vi "Button Lower Arm.vi"(7 "Description":string, 8 "Command Info In":T1, 9 "Deadband Value":dbl=0.01, 10 "Duration":dbl, 11 "Setpoint":dbl) -> (0 "Command Info Out":T1)   [LabVIEW 2017]
doc: "This template includes code for deadband comparision to avoid excessive command scheduling. It is particularly useful for joystick-driven commands.\n\nBe sure to right-click and select New from Template and save with a new command name."
uses:
  <vilib>/Rock Robotics/WPI/Framework/Command Status Info.ctl
  <vilib>/Rock Robotics/WPI/Framework/Completion Status.ctl
  <vilib>/Rock Robotics/WPI/Framework/Completion Notifier.ctl
  Implementation/Arm Setpoints.ctl
  Implementation/Arm Operations.ctl
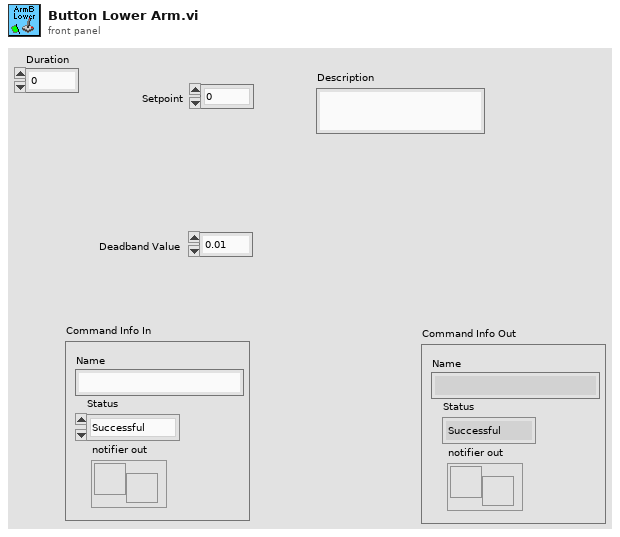
[diagram p1: front panel]
types:
  T1 = typedef "Command Status Info.ctl" = cluster{"Name":string, "Status":T2, "notifier out":T3}
  T2 = typedef "Completion Status.ctl" = enum16{"Successful", "Aborted", "Incomplete"}
  T3 = typedef "Completion Notifier.ctl" = refnum<notifier>
  T4 = typedef "Arm Setpoints.ctl" = cluster{"Operation":T5, "Setpoint":dbl, "Duration":dbl}
  T5 = typedef "Arm Operations.ctl" = enum16{"Reserve", "Read Current", "Immediate", "Lift Arm", "Lower Arm ", "Button Lift Arm", "Button Lower Arm"}
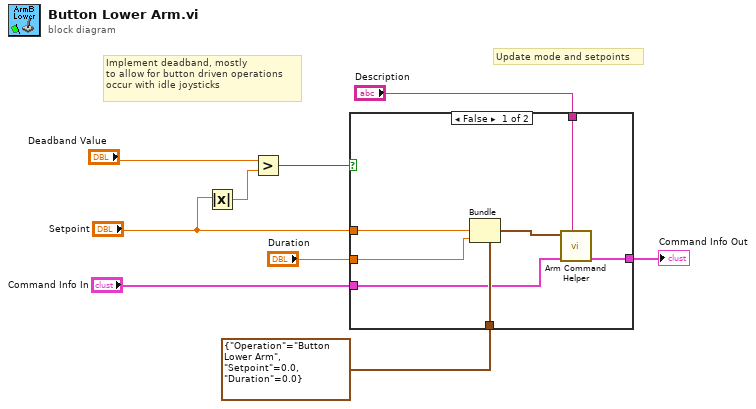
[diagram p0: block diagram]
diagram:
  # "Implement deadband, mostly\nto allow for button driven operations\noccur with idle joysticks"
  # "Update mode and setpoints"
  n1 = Absolute Value(x="Setpoint") -> (abs(x)=w8:dbl)
  n2 = Greater?(x="Deadband Value", y=w8) -> (0:w2:bool)
  n3 = case shown="False" w2 {
    tunnel: "Setpoint" -> [w16 _]
    tunnel: T4 {"Operation"=enum."Button Lower Arm", "Setpoint"=0.0, "Duration"=0.0} ("SubSystem Data") -> [w15 _]
    tunnel: [w14 w17] -> w7
    tunnel: "Command Info In" -> [w13 w17]
    tunnel: "Description" -> [w11 _]
    tunnel: "Duration" -> [w10 _]
    frame False {
      n4 = Bundle(cluster=w15, "Setpoint"=w16, "Duration"=w10) -> (w12:T4)  [unwired: 1 in]
      n5 = call "Arm Command Helper.vi"("Description"=w11, "Command Info In"=w13, "SubSystem Data"=w12) -> ("Command Info Out"=w14:T1)  [unwired: 6 in, 2 out]
    }
    frame True {
    }
  }
  "Command Info Out" <- w7
